vi "Create Callback Accessors.vi"(8 "Error In":errorcluster, 10 "Properties Folder":path, 11 "Class Path":path) -> (0 "Error Out":errorcluster)   [LabVIEW 2011, in "Generator.lvlib"]
doc: "This VI scripts the accessor VIs for every Callback of a class. It uses the BaseAccessorScriptor Class of the MemberVICreation.lvlib. It may be necessary to change accessscope of this library to run this VI."
uses:
  Generator.lvlib
  C:/Program Files (x86)/National Instruments/LabVIEW 2011/resource/Framework/Providers/LVClassLibrary/NewAccessors/BaseAccessorScripter/BaseAccessorScripter.lvclass
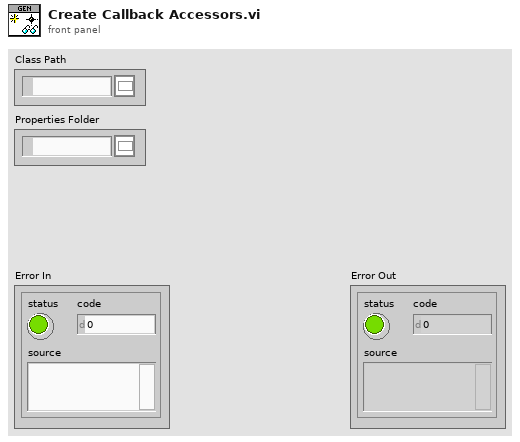
[diagram p1: front panel]
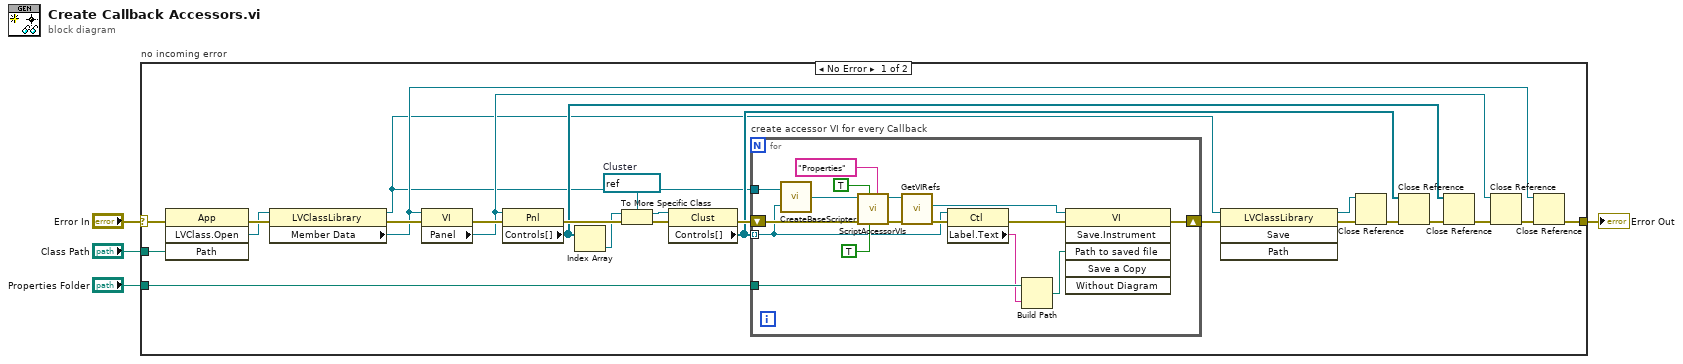
[diagram p0: block diagram]
diagram:
  n1 = case "no incoming error" shown="No Error" "Error In" {
    selector: "Error In" -> [w30 w47]
    tunnel: [w5 w47] -> w3
    tunnel: "Class Path" -> [w29 _]
    tunnel: "Properties Folder" -> [w19 _]
    frame No Error {
      w23 = refnum<vi> refnum  # Cluster
      n2 = invoke class="App" method="LVClass.Open"(error in=w30, "Path"=w29) -> (error out=w28:errorcluster, "LVClass.Open"=w7:refnum<vi>)  [unwired: 2 in, 2 out]
      n3 = property class="LVClassLibrary"(reference=w7, error in=w28) -> (reference out=w6:refnum<vi>, error out=w27:errorcluster, "Member Data"=w8:refnum<vi>)
      n4 = property class="VI"(reference=w8, error in=w27) -> (error out=w26:errorcluster, "Panel"=w9:refnum<vi>)  [unwired: 1 out]
      n5 = property class="Pnl"(reference=w9, error in=w26) -> (error out=w25:errorcluster, "Controls[]"=w12:refnum<vi>[])  [unwired: 1 out]
      n6 = Index Array(array=w12) -> (element=w24:refnum<vi>)  [unwired: 1 in]
      n7 = To More Specific Class(target class=w23, reference=w24, error in=w25) -> (specific class reference=w21:refnum<vi>, error out=w22:errorcluster)
      n8 = property class="Clust"(reference=w21, error in=w22) -> (error out=w20:errorcluster, "Controls[]"=w14:refnum<vi>[])  [unwired: 1 out]
      n9 = for "create accessor VI for every Callback" {
        shift-right: [w31] -> w18
        shift-left: w20 -> [w40]
        tunnel: w14 -> [w37] mode=indexing
        tunnel: w6 -> [w39]
        tunnel: w19 -> [w36]
        n10 = call "CreateBaseScripter.vi"("Ctl Refnum"=w37, "LVClassLibrary Ref"=w39) -> ("Scripter Out"=w46:refnum<class "BaseAccessorScripter.lvclass">)
        n11 = call-dynamic "ScriptAccessorVIs.vi"("Virtual Folder Name"="Properties", "Create as Properties"=TRUE, "Include error terminals"=TRUE, "error in (no error)"=w40, "BaseAccessorScripter in"=w46) -> ("error out"=w41:errorcluster, "BaseAccessorScripter out"=w42:refnum<class "BaseAccessorScripter.lvclass">)  [unwired: 5 in]
        n12 = call-dynamic "GetVIRefs.vi"("error in (no error)"=w41, "BaseAccessorScripter in"=w42) -> ("error out"=w38:errorcluster, "Read VI"=w33:refnum<vi>)  [unwired: 6 in, 2 out]
        n13 = property class="Ctl"(reference=w37, error in=w38) -> (error out=w34:errorcluster, "Label.Text"=w35:string)  [unwired: 1 out]
        n14 = Build Path(base path=w36, name or relative path=w35) -> (appended path=w32:path)
        n15 = invoke class="VI" method="Save.Instrument"(reference=w33, error in=w34, "Path to saved file"=w32) -> (error out=w31:errorcluster)  [unwired: 3 in, 5 out]
      }
      n16 = invoke class="LVClassLibrary" method="Save"(reference=w6, error in=w18) -> (reference out=w16:refnum<vi>, error out=w17:errorcluster)  [unwired: 2 in, 2 out]
      n17 = Close Reference(reference=w16, error in (no error)=w17) -> (error out=w15:errorcluster)
      n18 = Close Reference(reference=w14, error in (no error)=w15) -> (error out=w13:errorcluster)
      n19 = Close Reference(reference=w12, error in (no error)=w13) -> (error out=w10:errorcluster)
      n20 = Close Reference(reference=w9, error in (no error)=w10) -> (error out=w11:errorcluster)
      n21 = Close Reference(reference=w8, error in (no error)=w11) -> (error out=w5:errorcluster)
    }
    frame Error {
    }
  }
  "Error Out" <- w3
